vi "New Fixed SideMenu.vi"(8 "Error In":errorcluster) -> (0 "Error Out":errorcluster, 3 "Fixed SideMenu":refnum<class "SideMenu.lvclass">)   [LabVIEW 2021, in "Appearance Actor.lvlib" / "SideMenu.lvclass"]
uses:
  SideMenu.lvclass
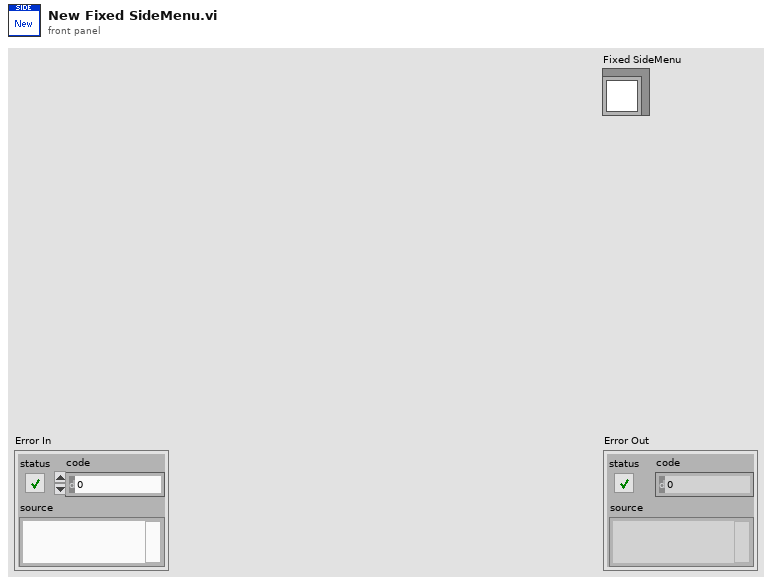
[diagram p1: front panel]
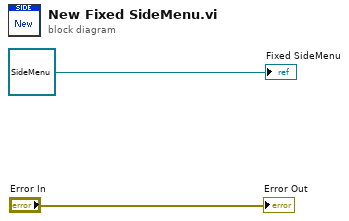
[diagram p0: block diagram]
diagram:
  "Error Out" <- "Error In"
  "Fixed SideMenu" <- refnum<class "SideMenu.lvclass"> refnum ("Fixed SideMenu")
